vi "_PluginLoader_GetPlugins.vi"(8 "error in (no error)":errorcluster, 11 "_PluginLoader in":refnum<class "_PluginLoader.lvclass">) -> (0 "error out":errorcluster, 2 "Plugins":refnum<class "GCMPlugin.lvclass">[](array[class]), 3 "_PluginLoader out":refnum<class "_PluginLoader.lvclass">)   [LabVIEW 2014, in "_PluginLoader.lvclass"]
uses:
  _PluginLoader.lvclass
  GCMPlugin/GCMPlugin.lvclass
  _PluginLoader.lvclass/_PluginLoader.ctl
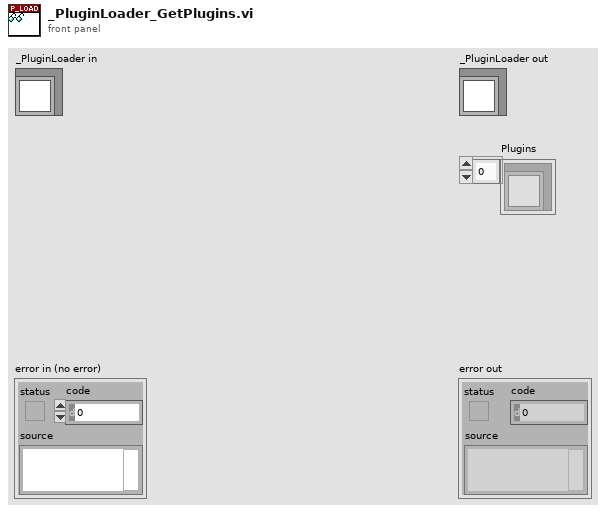
[diagram p1: front panel]
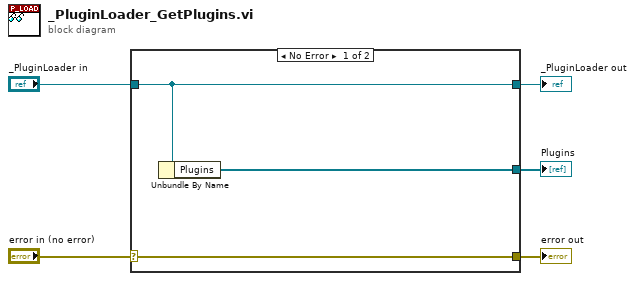
[diagram p0: block diagram]
diagram:
  n1 = case shown="No Error" "error in (no error)" {
    selector: "error in (no error)" -> [w8 w9]
    tunnel: [w8 w9] -> w4
    tunnel: [w7 w10] -> w2
    tunnel: "_PluginLoader in" -> [w7 w10]
    tunnel: [w6 _] -> w1
    frame No Error {
      n2 = Unbundle By Name(w7) -> ("Plugins"=w6:refnum<class "GCMPlugin.lvclass">[])
    }
    frame Error {
    }
  }
  "error out" <- w4
  "_PluginLoader out" <- w2
  "Plugins" <- w1
